vi "LoadPlugin.vi"(7 "reference":refnum<vi>, 8 "ErrorIn Array":errorcluster[](array[cluster]), 10 "Instrument Modules Old":T1=[{"PluginSelection"=4, "ConfigDialog"=FALSE}], 11 "Instrument Modules New In":T1=[{"PluginSelection"=4, "ConfigDialog"=FALSE}]) -> (0 "ErrorOut Array":errorcluster[](array[cluster]), 3 "Instrument Modules New Out":T1=[{"PluginSelection"=4, "ConfigDialog"=FALSE}])   [LabVIEW 2018]
doc: "This VI loads the new plugin into the module."
uses:
  Framework/InstrumentModulesControl.ctl
  NistPluggableModules/BusClass/Bus.lvclass/Bus.ctl
  NistPluggableModules/BusClass/Accessors/Write Test.vi
  NistPluggableModules/BusClass/Accessors/Read Test.vi
  NistPluggableModules/TestClass/Test.lvclass
  <userlib>/NIST/NISTErrorLib/NISTErrorLib.lvlib
  NistPluggableModules/BusClass/Bus.lvclass
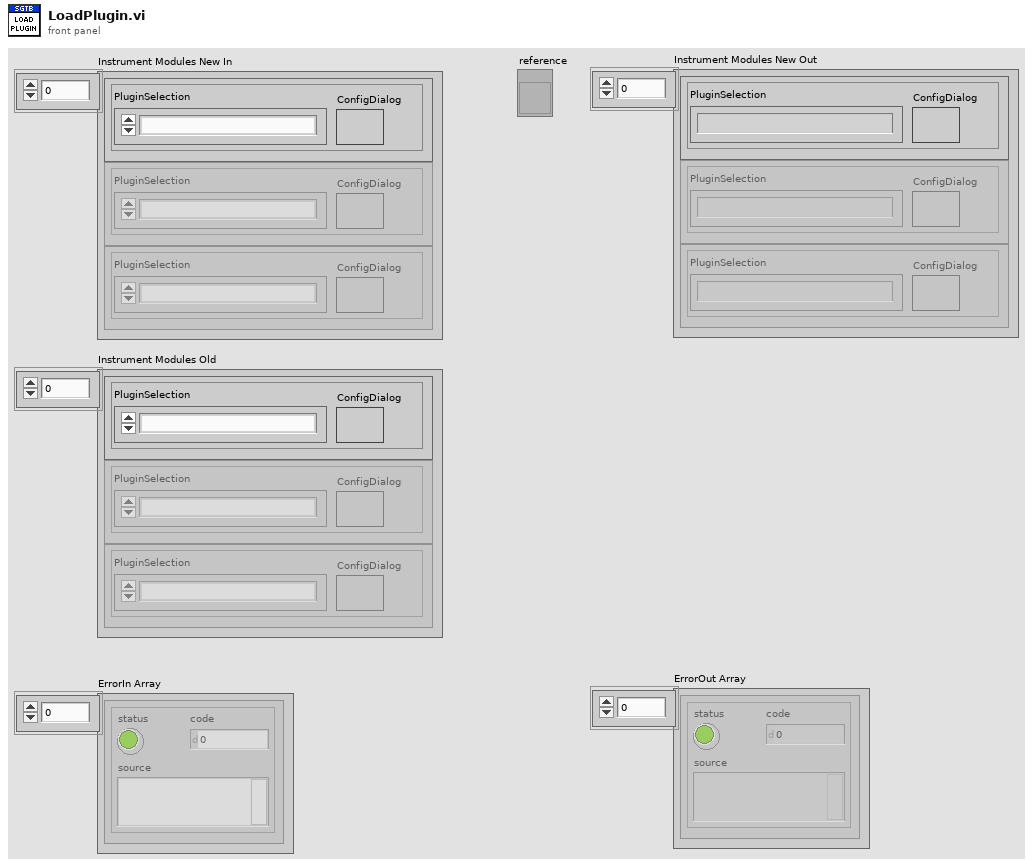
[diagram p1: front panel]
types:
  T1 = typedef "InstrumentModulesControl.ctl" = cluster{"PluginSelection":u16, "ConfigDialog":bool}[]
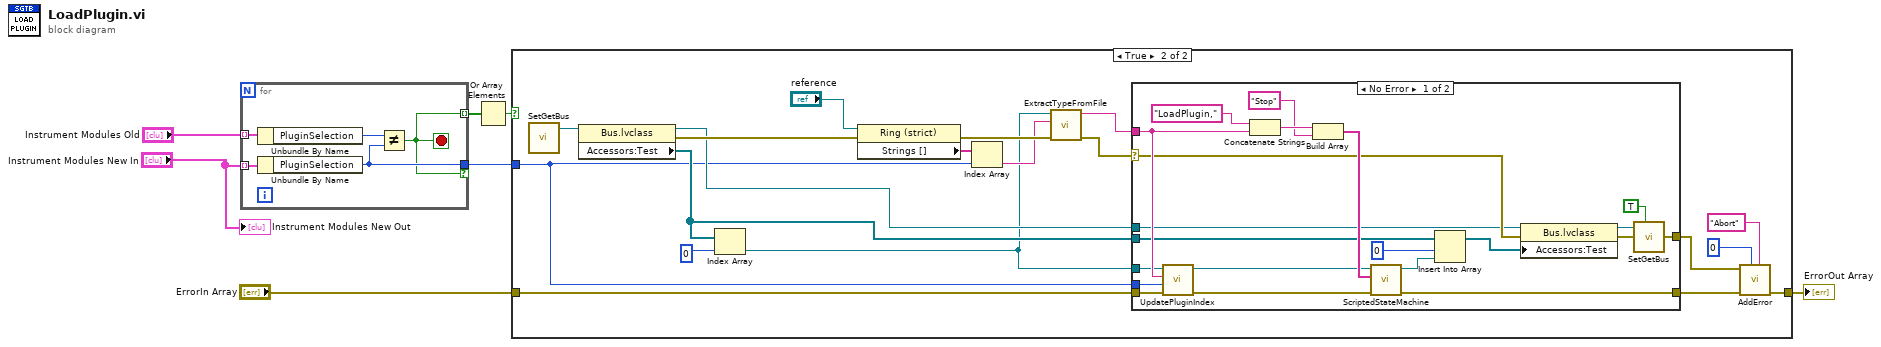
[diagram p0: block diagram]
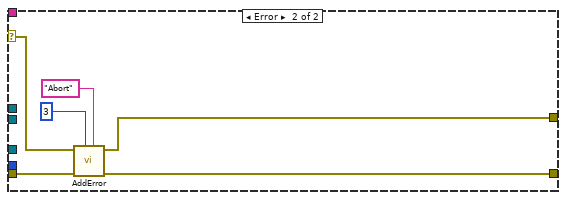
[diagram p3: hidden frame]
diagram:
  n1 = for {
    tunnel: "Instrument Modules New In" -> [w12] mode=indexing
    tunnel: "Instrument Modules Old" -> [w11] mode=indexing
    tunnel: [w9] -> w5 if=w8
    tunnel: [w8] -> w4 mode=indexing
    stop <- w8 stop-if-true
    n2 = Unbundle By Name(w11) -> ("PluginSelection"=w10:u16)
    n3 = Unbundle By Name(w12) -> ("PluginSelection"=w9:u16)
    n4 = Not Equal?(x=w10, y=w9) -> (x != y?=w8:bool)
  }
  n5 = Or Array Elements(Boolean array=w4) -> (logical OR=w3:bool)
  n6 = case shown="True" w3 {
    tunnel: "ErrorIn Array" -> [w13 w30]
    tunnel: [w13 w28] -> w6
    tunnel: w5 -> [_ w14]
    frame False {
    }
    frame True {
      n7 = call "SetGetBus.vi"() -> ("Bus.lvclass"=w26:refnum<class "Bus.lvclass">)  [unwired: 11 in]
      n8 = property class="Bus.lvclass"(reference=w26) -> (reference out=w18:refnum<class "Bus.lvclass">, error out=w21:errorcluster, "Accessors:Test"=w19:refnum<class "Test.lvclass">[])  [unwired: 1 in]
      n9 = Index Array(array=w19, index=0) -> (element=w17:refnum<class "Test.lvclass">)
      n10 = property class="Ring (strict)"(reference="reference", error in=w21) -> (error out=w23:errorcluster, "Strings []"=w24:string[])  [unwired: 1 out]
      n11 = Index Array(array=w24, index=w14) -> (element=w22:string)
      n12 = call "ExtractTypeFromFile.vi"("error in (no error)"=w23, "String"=w22, "Test in"=w17) -> ("error out"=w16:errorcluster, "Type"=w15:string)  [unwired: 7 in]
      n13 = case shown="No Error" w16 {
        selector: w16 -> [w42 w56]
        tunnel: w15 -> [w47 _]
        tunnel: [w52 w58] -> w27
        tunnel: w30 -> [w49 w57]
        tunnel: w14 -> [w48 _]
        tunnel: w17 -> [w46 _]
        tunnel: w19 -> [w41 _]
        tunnel: w18 -> [w37 _]
        tunnel: [w33 w53] -> w29
        frame No Error {
          n14 = call "UpdatePluginIndex.vi"("Error"=w49, "Index"=w48, "PluginName"=w47, "Test"=w46) -> ("Error"=w50:errorcluster[], "Test"=w45:refnum<class "Test.lvclass">)  [unwired: 6 in]
          n15 = Concatenate Strings("LoadPlugin," ("string"), w47) -> (w35:string)
          n16 = Build Array(w35, "Stop") -> (w51:string[])
          n17 = call "ScriptedStateMachine.vi"("ErrorArray"=w50, "script"=w51, "Test.lvclass"=w45) -> ("ErrorArray"=w52:errorcluster[], "Test.lvclass"=w40:refnum<class "Test.lvclass">)  [unwired: 6 in, 1 out]
          n18 = Insert Into Array(array=w41, index=0, new element=w40) -> (w39:refnum<class "Test.lvclass">[])
          n19 = property class="Bus.lvclass"(reference=w37, error in=w42, "Accessors:Test"=w39) -> (reference out=w38:refnum<class "Bus.lvclass">, error out=w33:errorcluster)
          n20 = call "SetGetBus.vi"("Set (f)"=TRUE, "Bus.lvclass"=w38) -> ()  [unwired: 9 in, 1 out]
        }
        frame Error {
          n21 = call <userlib>:"AddError.vi"("Severity"="Abort", "Priority"=u8 3, "ErrorArray"=w57, "error in (no error)"=w56) -> ("ErrorArray"=w58:errorcluster[], "error out"=w53:errorcluster)  [unwired: 6 in]
        }
      }
      n22 = call <userlib>:"AddError.vi"("Severity"="Abort", "Priority"=u8 0, "ErrorArray"=w27, "error in (no error)"=w29) -> ("ErrorArray"=w28:errorcluster[])  [unwired: 6 in, 1 out]
    }
  }
  "ErrorOut Array" <- w6
  "Instrument Modules New Out" <- "Instrument Modules New In"
